vi "test_trigger.vi"() -> (3 "test_result":T1)   [LabVIEW 2015]
uses:
  tester_result.ctl
  request/request.lvclass/request.ctl
  result/result.lvclass/result.ctl
  <vilib>/addons/lv-msgpack/MsgPack Deserializer/Unflatten From MessagePack.vi
  input/input.lvclass
  result/result.lvclass
  output/Output.lvclass
  request/request.lvclass
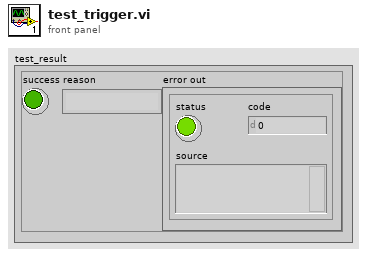
[diagram p1: front panel]
types:
  T1 = typedef "tester_result.ctl" = cluster{"success":bool, "reason":string, "error out":errorcluster}
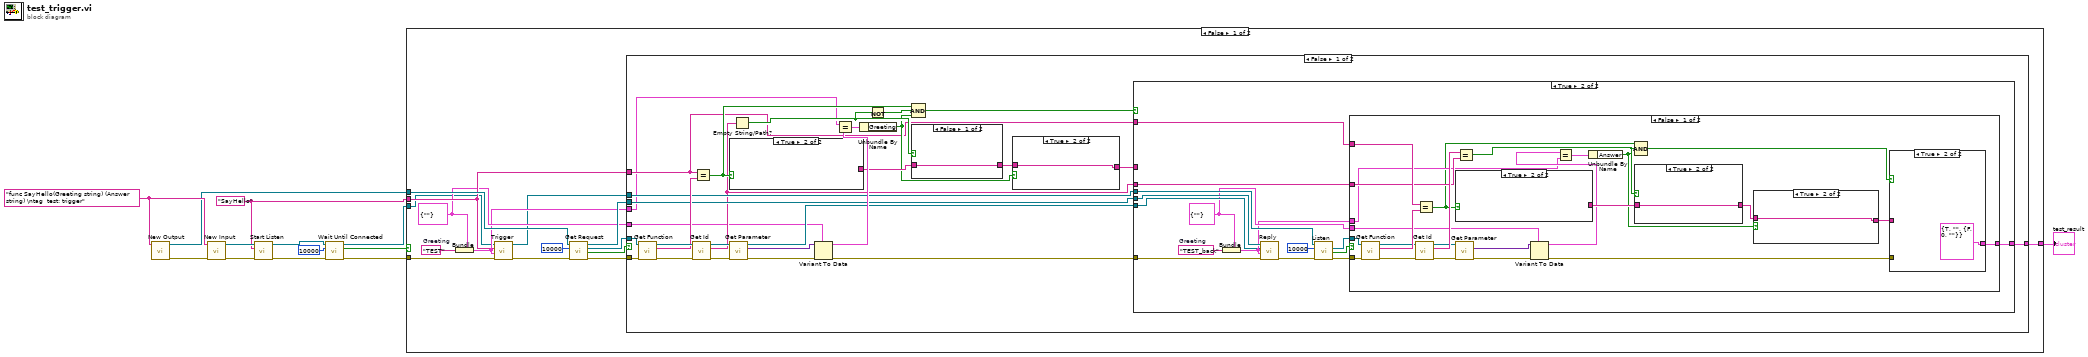
[diagram p0: block diagram]
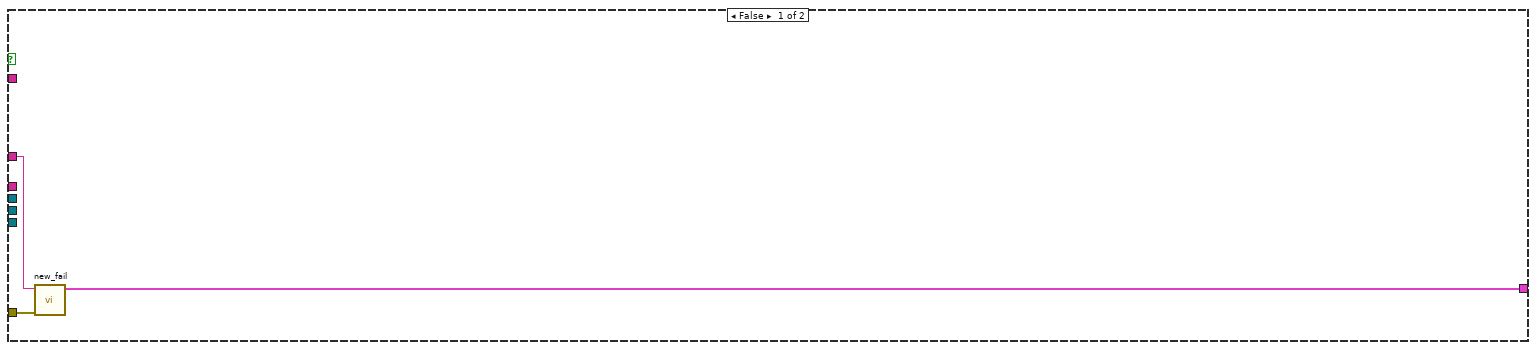
[diagram p2: hidden frame]
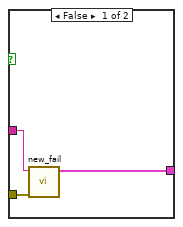
[diagram p3: hidden frame]
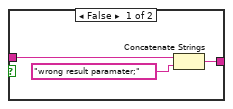
[diagram p4: hidden frame]
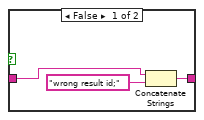
[diagram p5: hidden frame]
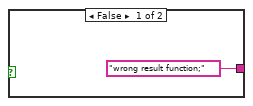
[diagram p6: hidden frame]
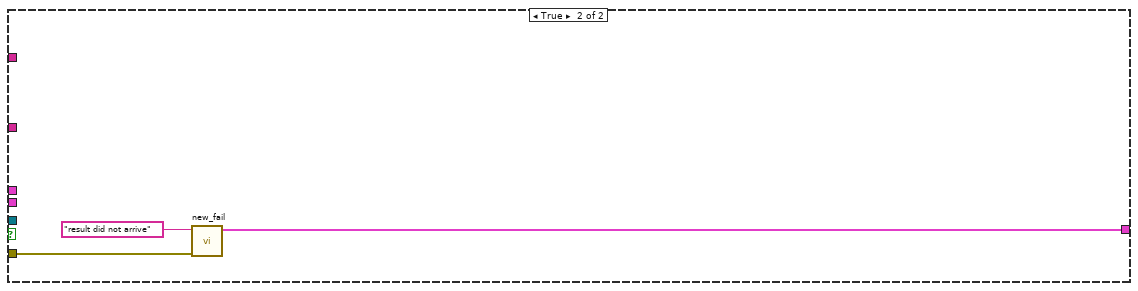
[diagram p7: hidden frame]
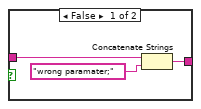
[diagram p8: hidden frame]
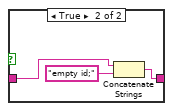
[diagram p9: hidden frame]
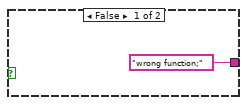
[diagram p10: hidden frame]
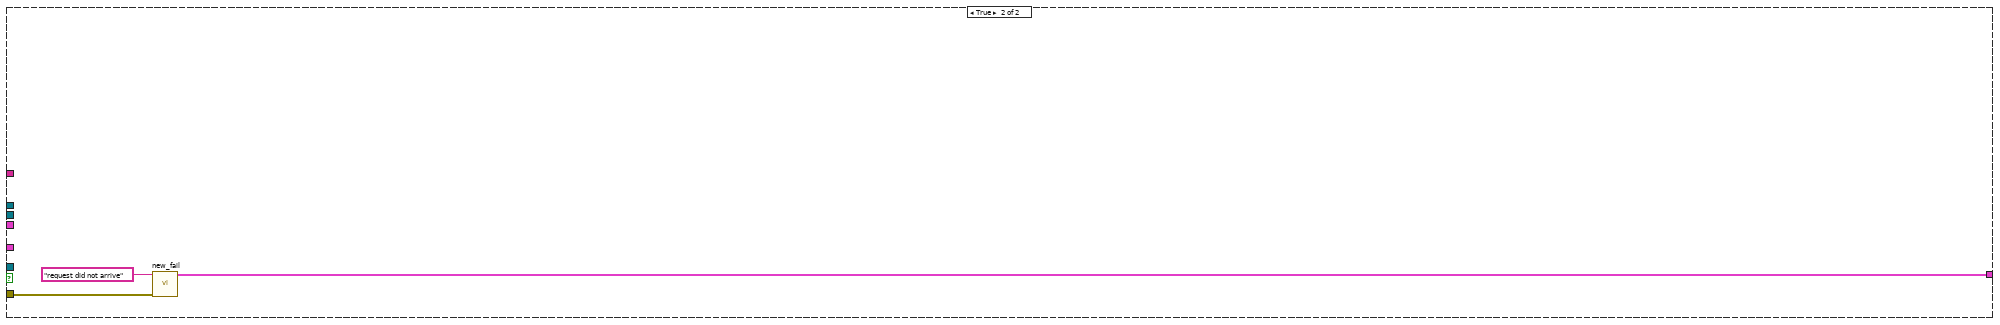
[diagram p11: hidden frame]
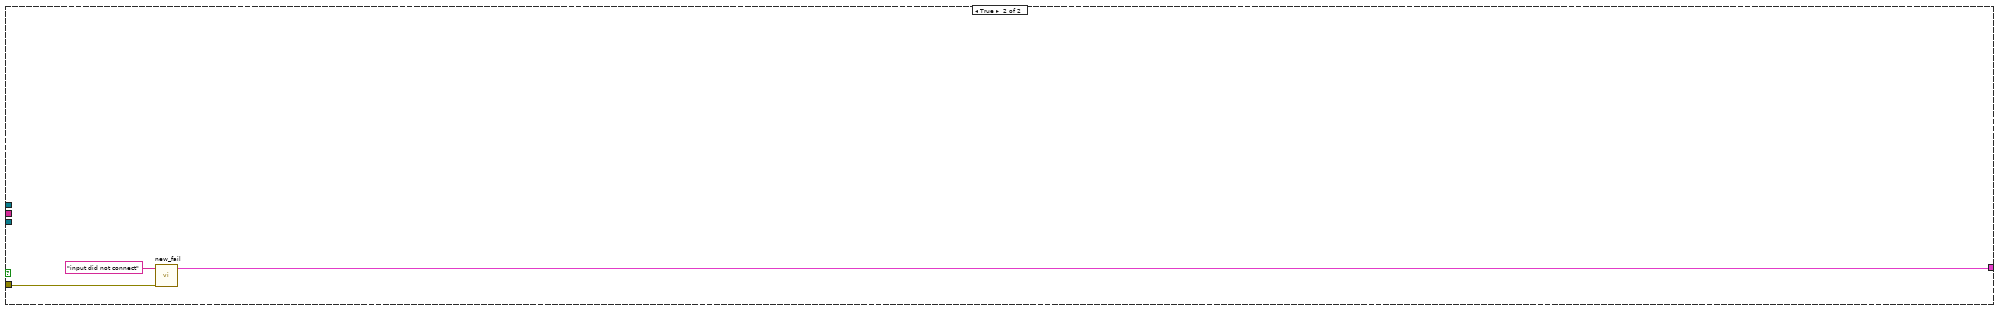
[diagram p12: hidden frame]
diagram:
  w7 = "SayHello" ("Function")
  w10 = "func SayHello(Greeting string) (Answer string) \ntag  test: trigger" ("Descriptor")
  n1 = call "New Output.vi"("Descriptor"=w10) -> ("error out"=w9:errorcluster, "output"=w8:refnum<class "Output.lvclass">)  [unwired: 9 in]
  n2 = call "New Input.vi"("error in (no error)"=w9, "Descriptor"=w10) -> ("error out"=w13:errorcluster, "input out"=w12:refnum<class "input.lvclass">)  [unwired: 8 in]
  n3 = call "Start Listen.vi"("error in (no error)"=w13, "Function"=w7, "input in"=w12) -> ("error out"=w5:errorcluster, "input out"=w6:refnum<class "input.lvclass">)  [unwired: 7 in]
  n4 = call "Wait Until Connected.vi"("error in (no error)"=w5, "timeout in ms (-1)"=10000, "input in"=w6) -> ("error out"=w4:errorcluster, "timeout"=w1:bool, "input out"=w3:refnum<class "input.lvclass">)  [unwired: 6 in]
  n5 = case shown="False" w1 {
    tunnel: [w28 w128] -> w11
    tunnel: w8 -> [w25 _]
    tunnel: w7 -> [w20 _]
    tunnel: w4 -> [w15 w130]
    tunnel: w3 -> [w14 _]
    frame False {
      w21 = "TEST"  # Greeting
      w19 = cluster{"Greeting":string} {"Greeting"=""}
      n6 = Bundle(cluster=w19, "Greeting"=w21) -> (w18:cluster{"Greeting":string})
      n7 = call "Trigger.vi"("error in (no error)"=w15, "Parameter"=w18, "Function"=w20, "input in"=w14) -> ("error out"=w27:errorcluster, "input out"=w16:refnum<class "input.lvclass">)  [unwired: 6 in]
      n8 = call "Get Request.vi"("error in (no error)"=w27, "timeout in ms (-1)"=10000, "output in"=w25) -> ("error out"=w26:errorcluster, "timed out?"=w24:bool, "request.lvclass"=w22:refnum<class "request.lvclass">, "output out"=w23:refnum<class "Output.lvclass">)  [unwired: 5 in]
      n9 = case shown="False" w24 {
        tunnel: [w56 w127] -> w28
        tunnel: w26 -> [w54 w126]
        tunnel: w23 -> [w35 _]
        tunnel: w22 -> [w55 _]
        tunnel: w20 -> [w32 _]
        tunnel: w19 -> [w30 _]
        tunnel: w18 -> [w29 _]
        tunnel: w16 -> [w33 _]
        frame False {
          n10 = call "Get Function.vi"("error in (no error)"=w54, "request in"=w55) -> ("error out"=w53:errorcluster, "function"=w49:string, "request out"=w51:refnum<class "request.lvclass">)  [unwired: 7 in]
          n11 = call "Get Id.vi"("error in (no error)"=w53, "request in"=w51) -> ("error out"=w52:errorcluster, "id"=w31:string, "request out"=w50:refnum<class "request.lvclass">)  [unwired: 7 in]
          n12 = Equal?(x=w32, y=w49) -> (x = y?=w41:bool)
          n13 = case shown="True" w41 {
            tunnel: ["wrong function;" ("source") _] -> w44
            frame False {
            }
            frame True {
            }
          }
          n14 = call "Get Parameter.vi"("error in (no error)"=w52, "request in"=w50) -> ("error out"=w48:errorcluster, "parameter"=w46:variant, "request out"=w34:refnum<class "request.lvclass">)  [unwired: 7 in]
          n15 = Empty String/Path?(string/path=w31) -> (empty?=w40:bool)
          n16 = Variant To Data(error in=w48, type=w30, Variant=w46) -> (data=w45:cluster{"Greeting":string}, error out=w47:errorcluster)
          n17 = Equal?(x=w29, y=w45) -> (x = y?=w42:cluster{"Greeting":bool})
          n18 = Unbundle By Name(w42) -> ("Greeting"=w38:bool)
          n19 = Not(x=w40) -> (.not. x?=w39:bool)
          n20 = Compound Arithmetic op=AND(w41, w39, w38) -> (w37:bool)
          n21 = case shown="False" w40 {
            tunnel: w44 -> [w120 w123]
            tunnel: [w120 w121] -> w43
            frame False {
            }
            frame True {
              n22 = Concatenate Strings(w123, "empty id;" ("source")) -> (w121:string)
            }
          }
          n23 = case shown="True" w38 {
            tunnel: w43 -> [w118 w119]
            tunnel: [w116 w119] -> w36
            frame False {
              n24 = Concatenate Strings(w118, "wrong paramater;" ("source")) -> (w116:string)
            }
            frame True {
            }
          }
          n25 = case shown="True" w37 {
            tunnel: [w58 w74] -> w56
            tunnel: w47 -> [w57 w73]
            tunnel: w36 -> [w59 _]
            tunnel: w35 -> [_ w72]
            tunnel: w34 -> [_ w71]
            tunnel: w33 -> [_ w69]
            tunnel: w32 -> [_ w64]
            tunnel: w31 -> [_ w62]
            frame False {
              n26 = call "new_fail.vi"("error out"=w57, "reason"=w59) -> ("result"=w58:T1)  [unwired: 9 in]
            }
            frame True {
              w70 = "TEST_back"  # Greeting
              w61 = cluster{"Answer":string} {"Answer"=""}
              n27 = Bundle(cluster=w61, "Answer"=w70) -> (w60:cluster{"Answer":string})
              n28 = call "Reply.vi"("error in (no error)"=w73, "parameter"=w60, "request"=w71, "output in"=w72) -> ("error out"=w68:errorcluster)  [unwired: 6 in, 1 out]
              n29 = call-dynamic "Listen.vi"("error in (no error)"=w68, "timeout in ms (-1)"=10000, "input in"=w69) -> ("error out"=w67:errorcluster, "timed out?"=w65:bool, "result"=w63:refnum<class "result.lvclass">)  [unwired: 5 in, 1 out]
              n30 = case shown="False" w65 {
                tunnel: [w99 w113] -> w74
                tunnel: w67 -> [w82 w114]
                tunnel: w64 -> [w98 _]
                tunnel: w63 -> [w97 _]
                tunnel: w62 -> [w92 _]
                tunnel: w61 -> [w86 _]
                tunnel: w60 -> [w84 _]
                frame False {
                  n31 = call "Get Function.vi"("error in (no error)"=w82, "result in"=w97) -> ("error out"=w91:errorcluster, "function"=w96:string, "result out"=w94:refnum<class "result.lvclass">)  [unwired: 7 in]
                  n32 = call "Get Id.vi"("error in (no error)"=w91, "result in"=w94) -> ("error out"=w90:errorcluster, "id"=w93:string, "result out"=w89:refnum<class "result.lvclass">)  [unwired: 7 in]
                  n33 = Equal?(x=w98, y=w96) -> (x = y?=w80:bool)
                  n34 = case shown="True" w80 {
                    tunnel: ["wrong result function;" ("source") _] -> w95
                    frame False {
                    }
                    frame True {
                    }
                  }
                  n35 = call-dynamic "Get Parameter.vi"("error in (no error)"=w90, "result in"=w89) -> ("error out"=w88:errorcluster, "Data"=w87:variant)  [unwired: 7 in, 1 out]
                  n36 = Equal?(x=w93, y=w92) -> (x = y?=w79:bool)
                  n37 = Variant To Data(error in=w88, type=w86, Variant=w87) -> (data=w85:cluster{"Answer":string}, error out=w81:errorcluster)
                  n38 = Equal?(x=w85, y=w84) -> (x = y?=w83:cluster{"Answer":bool})
                  n39 = Unbundle By Name(w83) -> ("Answer"=w75:bool)
                  n40 = Compound Arithmetic op=AND(w80, w79, w75) -> (w78:bool)
                  n41 = case shown="True" w79 {
                    tunnel: w95 -> [w110 w111]
                    tunnel: [w108 w111] -> w76
                    frame False {
                      n42 = Concatenate Strings(w110, "wrong result id;" ("source")) -> (w108:string)
                    }
                    frame True {
                    }
                  }
                  n43 = case shown="True" w75 {
                    tunnel: w76 -> [w106 w107]
                    tunnel: [w104 w107] -> w77
                    frame False {
                      n44 = Concatenate Strings(w106, "wrong result paramater;" ("source")) -> (w104:string)
                    }
                    frame True {
                    }
                  }
                  n45 = case shown="True" w78 {
                    tunnel: [w100 T1 {"success"=TRUE, "reason"="", "error out"={"status"=FALSE, "code"=0, "source"=""}} ("result")] -> w99
                    tunnel: w81 -> [w101 _]
                    tunnel: w77 -> [w102 _]
                    frame False {
                      n46 = call "new_fail.vi"("error out"=w101, "reason"=w102) -> ("result"=w100:T1)  [unwired: 9 in]
                    }
                    frame True {
                    }
                  }
                }
                frame True {
                  n47 = call "new_fail.vi"("error out"=w114, "reason"="result did not arrive") -> ("result"=w113:T1)  [unwired: 9 in]
                }
              }
            }
          }
        }
        frame True {
          n48 = call "new_fail.vi"("error out"=w126, "reason"="request did not arrive") -> ("result"=w127:T1)  [unwired: 9 in]
        }
      }
    }
    frame True {
      n49 = call "new_fail.vi"("error out"=w130, "reason"="input did not connect") -> ("result"=w128:T1)  [unwired: 9 in]
    }
  }
  "test_result" <- w11
